vi "CCD-Trigger-LSCI.vi"(0 "Frames/Seq":i32=12, 1 "Exposure Width (ms) in":T1=5.0 format="%#_9f", 3 "Blue Exposure Width [50-100] (ms)":T1=41.0 format="%#_9f", 4 "Time Between (ms)":T2=1.5 format="%#_9f", 5 "Red Start Time":T1=106.0 format="%#_9f", 7 "Sampling Rate":T1=100000.0 format="%#_9f", 8 "Amber Start Time":T1=53.0 format="%#_9f", 15 "Red Exposure Width [50-80] (ms)":T1=41.0 format="%#_9f", 17 "Amber Exposure Width [50-100] (ms)":T1=41.0 format="%#_9f", 19 "Delay End (ms)":T2=82.0 format="%#_9f") -> (2 "Blue LED":cluster{i32, dbl, dbl[]}(graph)={0, 1e-05, array[16000 elements]}, 6 "LSCI CCD":cluster{i32, dbl, dbl[]}(graph)={0, 1e-05, array[16000 elements]}, 9 "Amber LED":cluster{i32, dbl, dbl[]}(graph)={0, 1e-05, array[15900 elements]}, 10 "Whisker Cam":cluster{i32, dbl, dbl[]}(graph)={0, 1e-05, array[16000 elements]}, 11 "EMCCD Trigger":cluster{i32, dbl, dbl[]}(graph)={0, 1e-05, array[16000 elements]}, 12 "Array out":u32[](array[numeric]), 13 "Period (ms)":dbl=6.5, 14 "# Samples":T1=7800.0 format="%#_9f", 18 "Red LED":cluster{i32, dbl, dbl[]}(graph)={0, 1e-05, array[16000 elements]})   [LabVIEW 2021]
uses:
  Settings.ctl
  Control 2.ctl
  <vilib>/measure/NI_MABase.lvlib
panel:
  out "size(s) 2":i32=15900
  out "Trial On":cluster{i32, dbl, dbl[]}(graph)={0, 1e-05, array[16000 elements]}
  out "1 2":T1 format="%#_9f"
  out "1":T1 format="%#_9f"
  in  "index":i32
  out "Boolean array":bool[](array[boolean])=[TRUE, TRUE, TRUE, FALSE, FALSE, FALSE, TRUE, FALSE, FALSE, FALSE, FALSE, FALSE, FALSE, FALSE, FALSE, FALSE, FALSE, FALSE, FALSE, FALSE, FALSE, FALSE, FALSE, FALSE, FALSE, FALSE, FALSE, FALSE, FALSE, FALSE, FALSE, FALSE]
  out "size(s)":i32=15900
  out "total":cluster{i32, dbl, dbl[]}(graph)={0, 1e-05, array[15900 elements]}
  out "Number of Samples":dbl=7800.0
  # "If you want to create output in port0/line0:4 then select\nthe binary u32: 000000....1111"
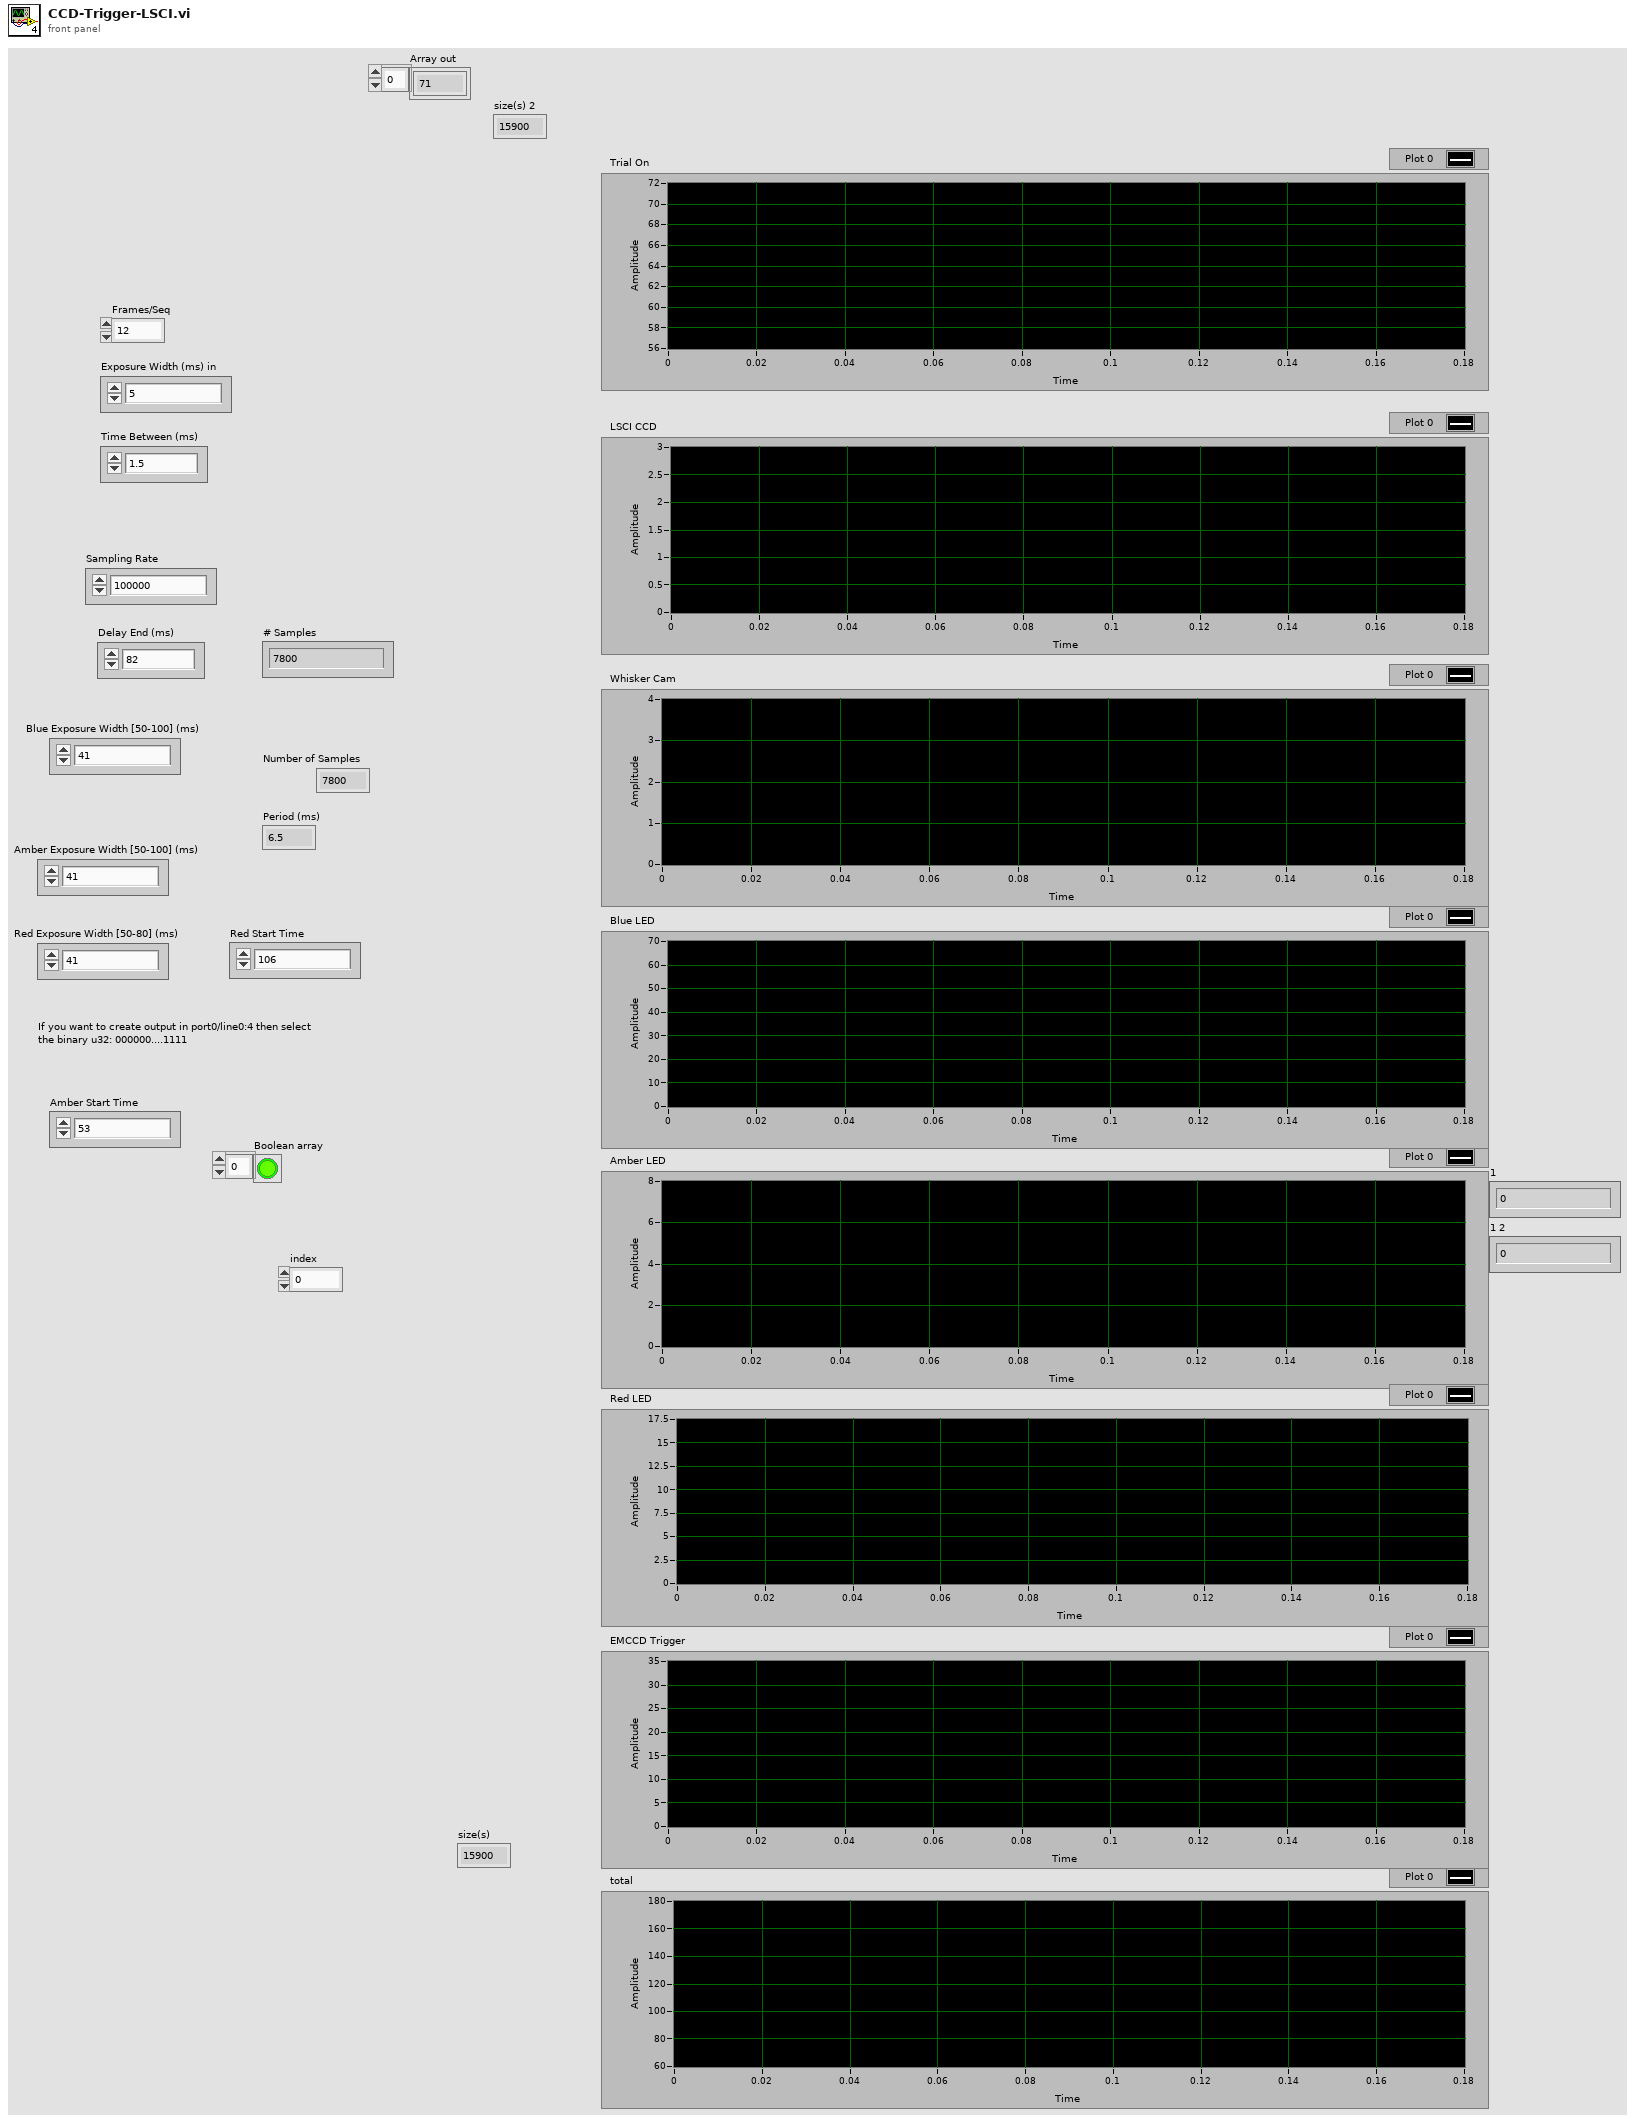
[diagram p1: front panel]
types:
  T1 = typedef "Settings.ctl" = dbl
  T2 = typedef "Control 2.ctl" = dbl
  T3 = cluster{"Sampling Rate":T1, "Exposure Width (ms) in":T1}
  T4 = cluster{"Sampling Rate":T1, "Amber Start Time":T1}
  T5 = cluster{"Sampling Rate":T1, "Amber Exposure Width [50-100] (ms) ":T1}
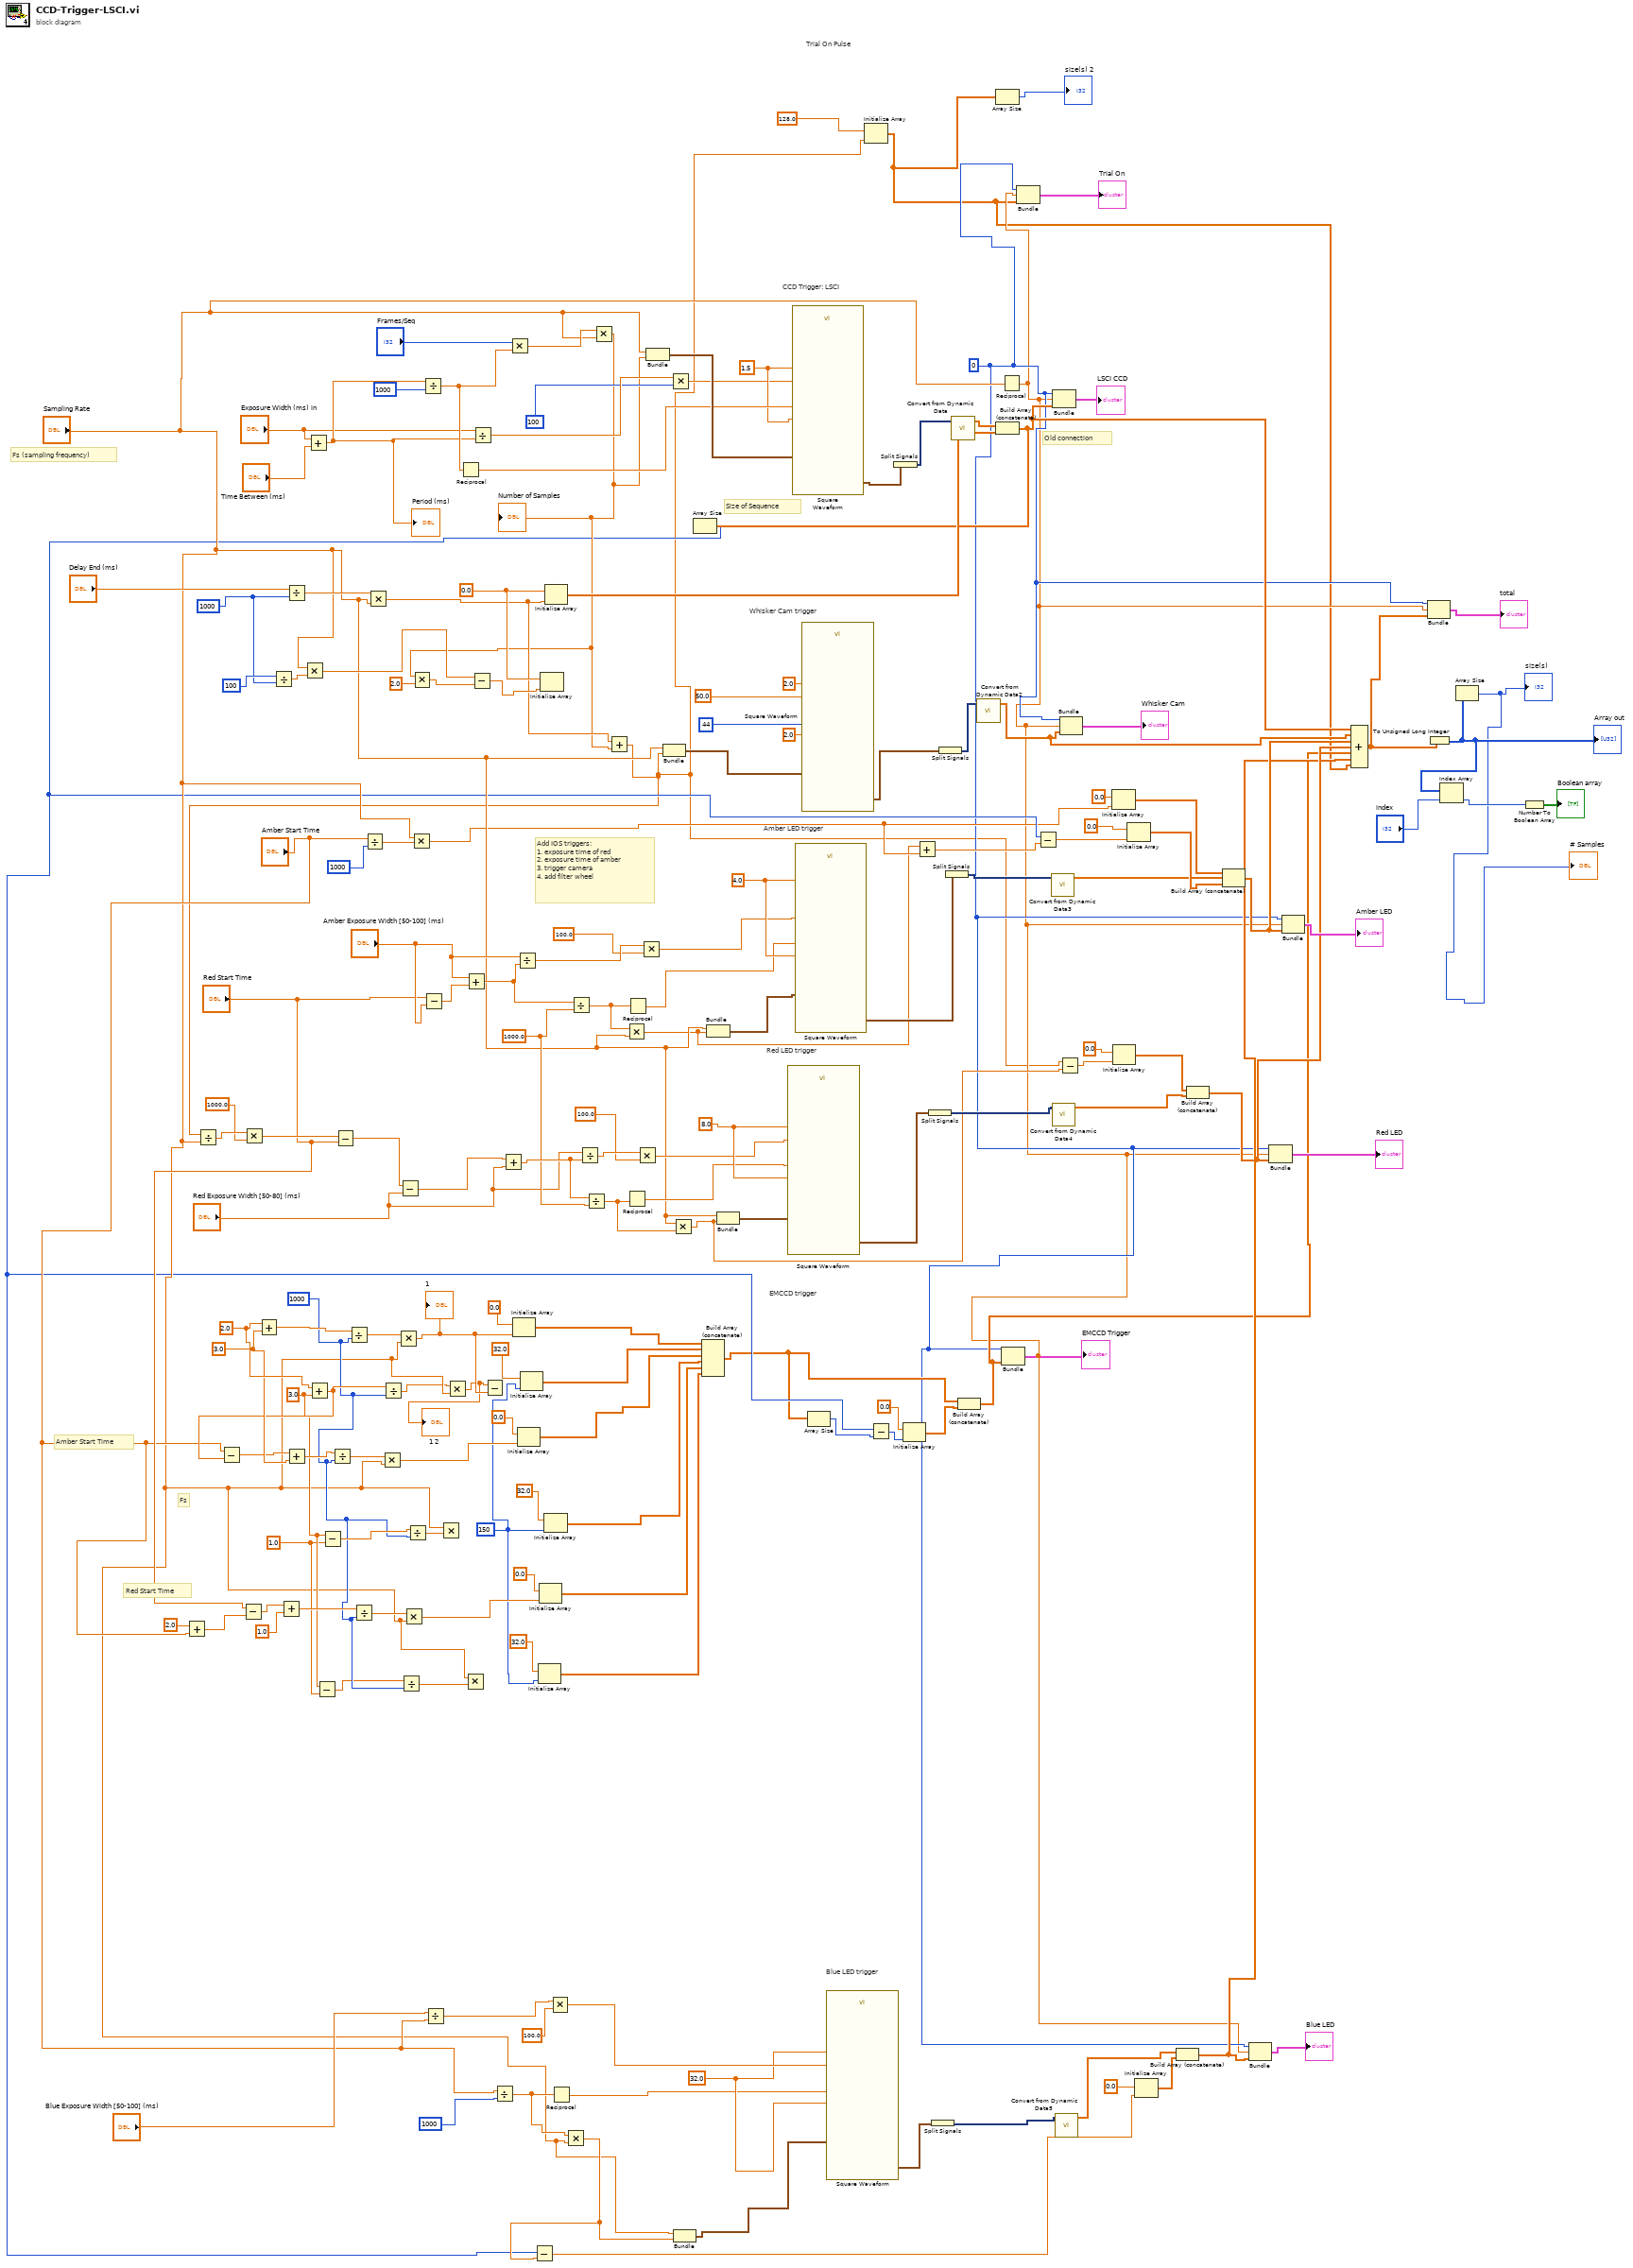
[diagram p0: block diagram]
diagram:
  w11 = 150 ("dimension size")
  w30 = 1.0 ("y")
  w33 = 1000
  w60 = 3.0 ("y")
  w31 = 3.0 ("y")
  w61 = 2.0 ("x")
  w74 = 32.0 ("element")
  w132 = 8.0 ("amplitude")
  w124 = T1 1000.0 ("y")
  w140 = 4.0 ("amplitude")
  w151 = 1000
  w147 = 0.0 ("element")
  w8 = 0
  w95 = 1.5
  # "Trial On Pulse"
  # "Fs"
  # "Size of Sequence"
  # "Red Start Time"
  # "Amber Start Time"
  # "Blue LED trigger"
  # "EMCCD trigger"
  # "Red LED trigger"
  # "Amber LED trigger"
  # "Whisker Cam trigger"
  # "Add IOS triggers:\n1. exposure time of red\n2. exposure time of amber\n3. trigger camera\n4. add filter wheel"
  # "Old connection"
  # "CCD Trigger: LSCI"
  # "Fs (sampling frequency)"
  n1 = Add(x=T1 2.0, y="Amber Start Time") -> (x+y=w39:T1)
  n2 = Subtract(x="Red Start Time", y=w39) -> (x-y=w38:T1)
  n3 = Add(x=w61, y=w60) -> (x+y=w62:dbl)
  n4 = Divide(x=100, y=w151) -> (x/y=w150:dbl)
  n5 = Add(x=w38, y=T1 1.0) -> (x+y=w36:T1)
  n6 = Divide(x="Delay End (ms)", y=w151) -> (x/y=w160:T2)
  n7 = Multiply(x="Sampling Rate", y=w150) -> (x*y=w149:T1)
  n8 = Add(x="Exposure Width (ms) in", y="Time Between (ms)") -> (x+y=w168:T1)
  "Period (ms)" <- w168
  n9 = Add(x=w61, y=w31) -> (x+y=w59:dbl)
  n10 = Subtract(x="Amber Start Time", y=w59) -> (x-y=w58:T1)
  n11 = Add(x=w58, y=w60) -> (x+y=w57:T1)
  n12 = Subtract(x=w31, y=w30) -> (x-y=w32:dbl)
  n13 = Subtract(x=w31, y=w30) -> (x-y=w47:dbl)
  n14 = Divide(x=w57, y=w33) -> (x/y=w56:T1)
  n15 = Divide(x=w62, y=w33) -> (x/y=w65:dbl)
  n16 = Divide(x=w36, y=w33) -> (x/y=w45:T1)
  n17 = Divide(x="Amber Start Time", y=1000) -> (x/y=w84:T1)
  n18 = Multiply(x=w160, y="Sampling Rate") -> (x*y=w141:T2)
  n19 = Multiply(x=w56, y="Sampling Rate") -> (x*y=w55:T1)
  n20 = Divide(x=w59, y=w33) -> (x/y=w14:dbl)
  n21 = Multiply(x=w65, y="Sampling Rate") -> (x*y=w51:T1)
  "1" <- w51
  n22 = Divide(x=w32, y=w33) -> (x/y=w34:dbl)
  n23 = Multiply(x=w45, y="Sampling Rate") -> (x*y=w44:T1)
  n24 = Divide(x=w47, y=w33) -> (x/y=w49:dbl)
  n25 = Multiply(x="Sampling Rate", y=w84) -> (x*y=w16:T1)
  n26 = Divide(x=w168, y=1000) -> (x/y=w169:T1)
  n27 = Subtract(x="Red Start Time", y="Amber Exposure Width [50-100] (ms)") -> (x-y=w130:T1)
  n28 = Divide(x="Blue Exposure Width [50-100] (ms)", y="Amber Start Time") -> (x/y=w79:T1)
  n29 = Multiply(x="Sampling Rate", y=w49) -> ()  [unwired: 1 out]
  n30 = Multiply(x=w14, y="Sampling Rate") -> (x*y=w12:T1)
  "1 2" <- w12
  n31 = Reciprocal(x=w169) -> (1/x=w134:T1)
  n32 = Multiply(x="Sampling Rate", y=w34) -> ()  [unwired: 1 out]
  n33 = Add(x="Amber Exposure Width [50-100] (ms)", y=w130) -> (x+y=w133:T1)
  n34 = Divide(x="Exposure Width (ms) in", y=w168) -> (x/y=w164:T1)
  n35 = Subtract(x=w12, y=w51) -> ()  [unwired: 1 out]
  n36 = Divide(x="Amber Start Time", y=1000) -> (x/y=w76:T1)
  n37 = Multiply(x="Frames/Seq", y=w169) -> (x*y=w166:T1)
  n38 = Initialize Array(0.0 ("element"), w51) -> (w54:dbl[])
  n39 = Divide(x="Amber Exposure Width [50-100] (ms)", y=w133) -> (x/y=w139:T1)
  n40 = Initialize Array(0.0 ("element"), w55) -> (w52:dbl[])
  n41 = Initialize Array(32.0 ("element"), w11) -> (w53:dbl[])
  n42 = Initialize Array(32.0 ("element"), w11) -> (w29:dbl[])
  n43 = Initialize Array(0.0 ("element"), w44) -> (w43:dbl[])
  n44 = Initialize Array(32.0 ("element"), w11) -> (w48:dbl[])
  n45 = Initialize Array(w147, w141) -> (w143:dbl[])
  n46 = Multiply(x=w79, y=T1 100.0) -> (x*y=w78:T1)
  n47 = Reciprocal(x=w76) -> (1/x=w13:T1)
  n48 = Multiply(x=w76, y="Sampling Rate") -> (x*y=w27:T1)
  n49 = Divide(x=w133, y=w124) -> (x/y=w121:T1)
  n50 = Multiply(x=w166, y="Sampling Rate") -> (x*y=w82:T1)
  "Number of Samples" <- w82
  n51 = Multiply(x=w82, y=T1 2.0) -> (x*y=w148:T1)
  n52 = Subtract(x=w149, y=w148) -> (x-y=w146:T1)
  n53 = Initialize Array(w147, w146) -> ()  [unwired: 1 out]
  n54 = Add(x=w141, y=w82) -> (x+y=w4:T2)
  n55 = Divide(x=w4, y="Sampling Rate") -> (x/y=w106:T2)
  n56 = Multiply(x=w106, y=T2 1000.0) -> (x*y=w104:T2)
  n57 = Subtract(x=w104, y="Red Start Time") -> (x-y=w103:T2)
  n58 = Subtract(x=w103, y="Red Exposure Width [50-80] (ms)") -> (x-y=w129:T2)
  n59 = Add(x=w129, y="Red Exposure Width [50-80] (ms)") -> (x+y=w125:T2)
  n60 = Divide(x="Red Exposure Width [50-80] (ms)", y=w125) -> (x/y=w128:T1)
  n61 = Divide(x=w125, y=w124) -> (x/y=w120:T2)
  n62 = Multiply(x=w121, y="Sampling Rate") -> (x*y=w3:T1)
  n63 = Reciprocal(x=w120) -> (1/x=w123:T2)
  n64 = Reciprocal(x=w121) -> (1/x=w135:T1)
  n65 = Multiply(x=w128, y=T1 100.0) -> (x*y=w126:T1)
  n66 = Multiply(x=w139, y=T1 100.0) -> (x*y=w137:T1)
  n67 = Bundle("Sampling Rate"="Sampling Rate", "Exposure Width (ms) in"=w82) -> (w157:T3)  [unwired: 1 in]
  n68 = Bundle("Sampling Rate"="Sampling Rate", "Delay End (ms)"=w4) -> (w10:cluster{"Sampling Rate":T1, "Delay End (ms)":T2})  [unwired: 1 in]
  n69 = Multiply(x=w164, y=100) -> (x*y=w91:T1)
  n70 = Multiply(x="Sampling Rate", y=w120) -> (x*y=w107:T1)
  n71 = Bundle("Sampling Rate"="Sampling Rate", "Amber Start Time"=w27) -> (w75:T4)  [unwired: 1 in]
  n72 = Build Array (concatenate)(w54, w53, w52, w48, w43, w29) -> (w18:dbl[])
  n73 = Bundle("Sampling Rate"="Sampling Rate", "Amber Exposure Width [50-100] (ms)"=w3) -> (w131:T5)  [unwired: 1 in]
  n74 = Bundle("Sampling Rate"="Sampling Rate", "Sampling Rate"=w107) -> (w122:cluster{"Sampling Rate":T1, "Sampling Rate":T1})  [unwired: 1 in]
  n75 = call <vilib>:"Square Waveform.vi"("duty cycle (%)"=w126, "offset"=w132, "sampling info"=w122, "amplitude"=w132, "frequency"=w123) -> ("signal out"=w110:waveform(dbl))  [unwired: 5 in, 1 out]
  n76 = call <vilib>:"Square Waveform.vi"("duty cycle (%)"=w91, "offset"=w95, "sampling info"=w157, "amplitude"=w95, "frequency"=w134) -> ("signal out"=w170:waveform(dbl))  [unwired: 5 in, 1 out]
  n77 = call <vilib>:"Square Waveform.vi"("duty cycle (%)"=w137, "offset"=w140, "sampling info"=w131, "amplitude"=w140, "frequency"=w135) -> ("signal out"=w116:waveform(dbl))  [unwired: 5 in, 1 out]
  n78 = call <vilib>:"Square Waveform.vi"("duty cycle (%)"=50.0, "offset"=2.0, "sampling info"=w10, "amplitude"=2.0, "frequency"=44) -> ("signal out"=w155:waveform(dbl))  [unwired: 5 in, 1 out]
  n79 = Array Size(array=w18) -> (size(s)=w22:i32)
  n80 = call <vilib>:"Square Waveform.vi"("duty cycle (%)"=w78, "offset"=w74, "sampling info"=w75, "amplitude"=w74, "frequency"=w13) -> ("signal out"=w73:waveform(dbl))  [unwired: 5 in, 1 out]
  n81 = Initialize Array(128.0 ("amplitude"), w4) -> (w2:dbl[])
  n82 = Split Signals(w170) -> (w171:dynamicdata)  [unwired: 1 in]
  n83 = Add(x=w3, y=w16) -> (x+y=w15:T1)
  n84 = Split Signals(w110) -> (w111:dynamicdata)  [unwired: 1 in]
  n85 = Split Signals(w73) -> (w72:dynamicdata)  [unwired: 1 in]
  n86 = Split Signals(w155) -> (w154:dynamicdata)  [unwired: 1 in]
  n87 = Split Signals(w116) -> (w115:dynamicdata)  [unwired: 1 in]
  n88 = call "Convert from Dynamic Data"("Dynamic Data Type"=w171) -> ("Array"=w156:dbl[])  [unwired: 3 in]
  n89 = call "Convert from Dynamic Data2"("Dynamic Data Type"=w154) -> ("Array"=w94:dbl[])  [unwired: 3 in]
  n90 = Array Size(array=w2) -> (size(s)=→"size(s) 2":i32)
  n91 = Build Array (concatenate)(w156, w143) -> (w28:dbl[])
  n92 = Array Size(array=w28) -> (size(s)=w23:i32)
  n93 = Subtract(x=w23, y=w27) -> (x-y=w26:T1)
  n94 = Subtract(x=w23, y=w22) -> (x-y=w21:i32)
  n95 = Initialize Array(0.0 ("element"), w21) -> (w19:dbl[])
  n96 = Build Array (concatenate)(w18, w19) -> (w17:dbl[])
  n97 = Reciprocal(x="Sampling Rate") -> (1/x=w7:T1)
  n98 = Bundle(w8, w7, w17) -> (→"EMCCD Trigger":cluster{i32, T1, dbl[]})  [unwired: 1 in]
  n99 = Bundle(w8, w7, w2) -> (→"Trial On":cluster{i32, T1, dbl[]})  [unwired: 1 in]
  n100 = Subtract(x=w23, y=w15) -> (x-y=w24:T1)
  n101 = call "Convert from Dynamic Data3"("Dynamic Data Type"=w115) -> ("Array"=w114:dbl[])  [unwired: 3 in]
  n102 = call "Convert from Dynamic Data4"("Dynamic Data Type"=w111) -> ("Array"=w108:dbl[])  [unwired: 3 in]
  n103 = Bundle(w8, w7, w28) -> (→"LSCI CCD":cluster{i32, T1, dbl[]})  [unwired: 1 in]
  n104 = call "Convert from Dynamic Data5"("Dynamic Data Type"=w72) -> ("Array"=w70:dbl[])  [unwired: 3 in]
  n105 = Subtract(x=w4, y=w107) -> (x-y=w112:T2)
  n106 = Bundle(w8, w7, "Array"=w94) -> (→"Whisker Cam":cluster{i32, T1, "Array":dbl[]})  [unwired: 1 in]
  n107 = Initialize Array(0.0 ("element"), w16) -> (w83:dbl[])
  n108 = Initialize Array(0.0 ("element"), w112) -> (w109:dbl[])
  n109 = Initialize Array(0.0 ("element"), w24) -> (w117:dbl[])
  n110 = Initialize Array(0.0 ("element"), w26) -> (w69:dbl[])
  n111 = Build Array (concatenate)(w70, w69) -> (w67:dbl[])
  n112 = Build Array (concatenate)(w109, w108) -> (w102:dbl[])
  n113 = Build Array (concatenate)(w83, w114, w117) -> (w96:dbl[])
  n114 = Bundle(w8, w7, w67) -> (→"Blue LED":cluster{i32, T1, dbl[]})  [unwired: 1 in]
  n115 = Bundle(w8, w7, w102) -> (→"Red LED":cluster{i32, T1, dbl[]})  [unwired: 1 in]
  n116 = Bundle(w8, w7, w96) -> (→"Amber LED":cluster{i32, T1, dbl[]})  [unwired: 1 in]
  n117 = Compound Arithmetic op=ADD(w28, w94, w96, w102, w17, w67, w2) -> (w93:dbl[])
  n118 = Bundle(w8, w7, w93) -> (→"total":cluster{i32, T1, dbl[]})  [unwired: 1 in]
  n119 = To Unsigned Long Integer(number=w93) -> (unsigned 32bit integer=w100:u32[])
  "Array out" <- w100
  n120 = Index Array(array=w100, index="index") -> (element=w99:u32)
  n121 = Array Size(array=w100) -> (size(s)=→"# Samples" →"size(s)":i32)
  n122 = Number To Boolean Array(number=w99) -> (Boolean array=→"Boolean array":bool[])
